vi "Calibrate pH Sensor.vi"(6 "Initialize/Close?":bool, 7 "Calibration Standard":dbl, 8 "Error In (No Error)":errorcluster, 9 "Calibrate":bool=TRUE, 10 "Sensor Address In":string="0", 11 "RS232 Port In":refnum<visa-resource-name>="COM11") -> (0 "Error Out":errorcluster, 1 "Sensor Calibrate Response":bool, 2 "Address Out":string, 3 "RS232 Port Out":refnum<visa-resource-name>)   [LabVIEW 2016]
doc: "Sends an SDI-12 Send Identification Command, and returns the various attributes from the sensor's response.\n\nThe total size by the sensor must be 22-35 in size (inclusive), or this VI will return an error."
uses:
  SDI-12.lvlib
panel:
  out "read buffer":string
  out "output 1":i16
  out "Command":string
  # "(c) 2008 National Instruments.  ALL RIGHTS RESERVED."
  # "The following are required,\nor are optional, for the sensors\nto respond with:"
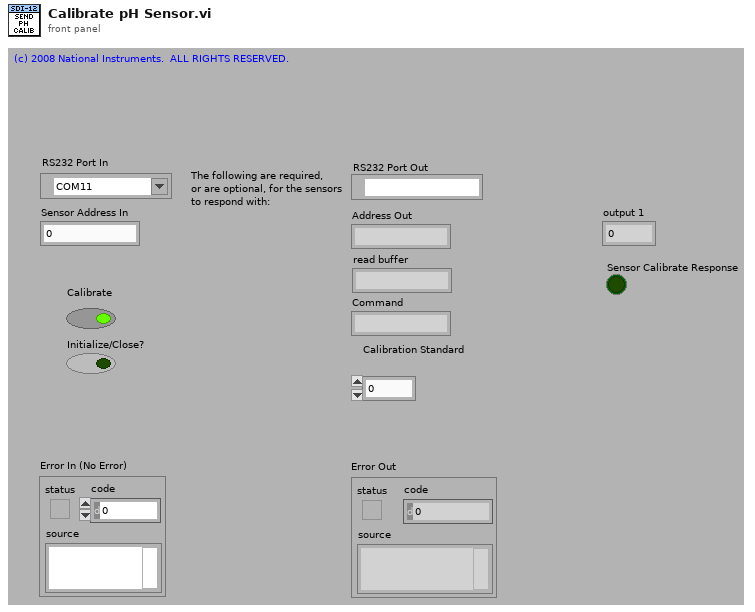
[diagram p1: front panel]
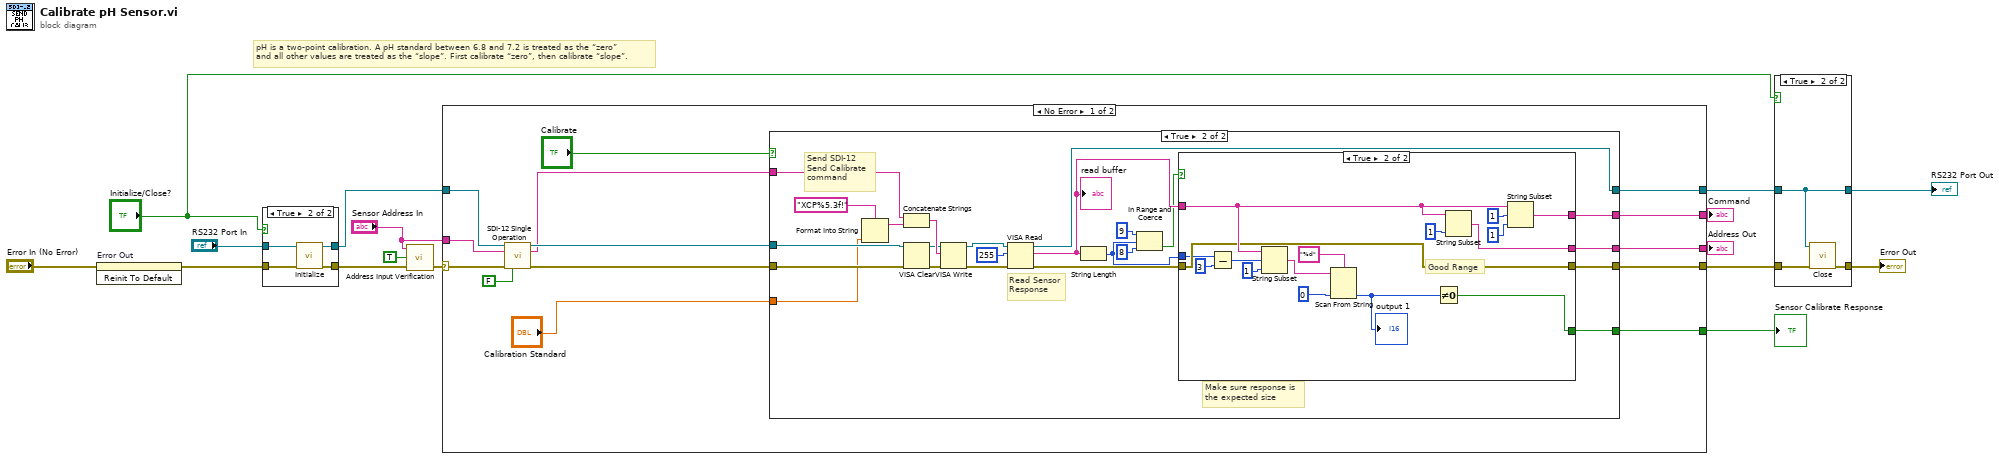
[diagram p0: block diagram]
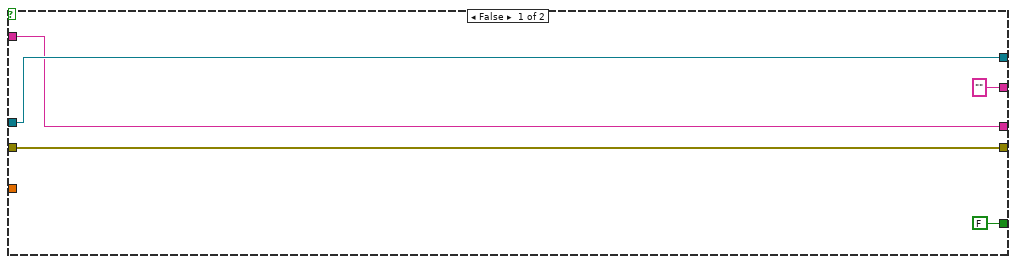
[diagram p4: hidden frame]
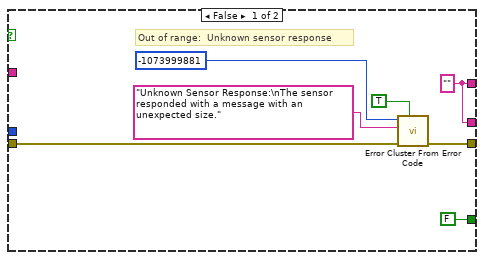
[diagram p5: hidden frame]
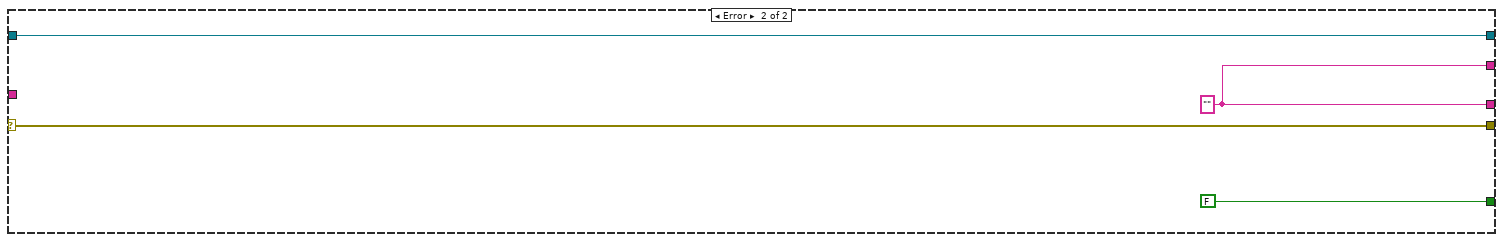
[diagram p6: hidden frame]
diagram:
  # "pH is a two-point calibration. A pH standard between 6.8 and 7.2 is treated as the “zero”\nand all other values are treated as the “slope”. First calibrate “zero”, then calibrate “slope”."
  n1 = invoke on="Error Out" class="Clust (strict)" method="Reinit To Default"(error in="Error In (No Error)") -> (error out=w1:errorcluster)  [unwired: 2 in, 2 out]
  n2 = case shown="True" "Initialize/Close?" {
    tunnel: w1 -> [w18 w22]
    tunnel: [w18 w21] -> w6
    tunnel: "RS232 Port In" -> [w17 w20]
    tunnel: [w17 w19] -> w4
    frame False {
    }
    frame True {
      n3 = call "Initialize.vi"("Error In (No Error)"=w22, "RS232 Port In"=w20) -> ("Error Out"=w21:errorcluster, "RS232 Port Out"=w19:refnum<visa-resource-name>)  [unwired: 8 in]
    }
  }
  n4 = call "Address Input Verification.vi"("Error In (No Error)"=w6, "Error if Bad? (True)"=TRUE ("error if bad? (True)"), "Sensor Address In (a)"="Sensor Address In") -> ("Error Out"=w16:errorcluster)  [unwired: 1 in, 1 out]
  n5 = case shown="No Error" w16 {
    selector: w16 -> [w30 w91]
    tunnel: [w35 w91] -> w10
    tunnel: "Sensor Address In" -> [w26 _]
    tunnel: w4 -> [w28 w90]
    tunnel: [w36 w90] -> w7
    tunnel: [w34 w89] -> w12
    tunnel: [w33 w89] -> w13
    tunnel: [w32 FALSE] -> w11
    frame No Error {
      n6 = call "SDI-12 Single Operation.vi"("RS232 Port In"=w28, "Sensor Address In"=w26, "Error In (No Error)"=w30, "Initialize/Close?"=FALSE) -> ("RS232 Port Out"=w27:refnum<visa-resource-name>, "Address Out"=w25:string, "Error Out"=w29:errorcluster)  [unwired: 7 in, 2 out]
      n7 = case shown="True" "Calibrate" {
        tunnel: w25 -> [w39 w61]
        tunnel: w27 -> [w41 w59]
        tunnel: [w41 w58] -> w36
        tunnel: [w40 w52] -> w35
        tunnel: ["" ("read buffer") w51] -> w34
        tunnel: [w39 w50] -> w33
        tunnel: [FALSE w47] -> w32
        tunnel: w29 -> [w40 w45]
        tunnel: "Calibration Standard" -> [_ w42]
        frame False {
        }
        frame True {
          # "Make sure response is\nthe expected size"
          # "Send SDI-12 \nSend Calibrate \ncommand"
          # "Read Sensor\nResponse"
          n8 = Format Into String(format string="XCP%5.3f!", w42) -> (resulting string=w48:string)  [unwired: 2 in, 1 out]
          n9 = Concatenate Strings(w61, w48) -> (w60:string)
          n10 = VISA Clear(VISA resource name=w59, error in (no error)=w45) -> (VISA resource name out=w46:refnum<visa-resource-name>, error out=w44:errorcluster)
          n11 = VISA Write(VISA resource name=w46, write buffer=w60, error in (no error)=w44) -> (VISA resource name out=w64:refnum<visa-resource-name>, error out=w63:errorcluster)  [unwired: 1 out]
          n12 = VISA Read(VISA resource name=w64, byte count=u32 255, error in (no error)=w63) -> (VISA resource name out=w58:refnum<visa-resource-name>, read buffer=w54:string, error out=w55:errorcluster)  [unwired: 1 out]
          "read buffer" <- w54
          n13 = String Length(string=w54) -> (length=w43:i32)
          n14 = In Range and Coerce(upper limit=9, x=w43, lower limit=8) -> (In Range?=w53:bool)  [unwired: 1 out]
          n15 = case shown="True" w53 {
            tunnel: w55 -> [w67 w82]
            tunnel: [w68 w82] -> w52
            tunnel: w54 -> [_ w84]
            tunnel: [w66 w80] -> w51
            tunnel: [w66 w79] -> w50
            tunnel: [FALSE w75] -> w47
            tunnel: w43 -> [_ w74]
            frame False {
              w66 = "" ("read buffer")
              # "Out of range:  Unknown sensor response"
              n16 = call <vilib>:"Error Cluster From Error Code.vi"("show call chain? (False)"=TRUE, "error in (no error)"=w67, "error message (\"\")"="Unknown Sensor Response:\nThe sensor responded with a message with an unexpected size." ("error message (\"\")"), "error code (0)"=-1073999881) -> ("error out"=w68:errorcluster)  [unwired: 5 in]
            }
            frame True {
              # "Good Range"
              n17 = Subtract(x=w74, y=3) -> (x-y=w73:i32)
              n18 = String Subset(string=w84, offset (0)=w73, length (rest)=1 ("length (rest)")) -> (substring=w81:string)
              n19 = Scan From String(format string="%d", input string=w81, default 1=i16 0 ("default value 1")) -> (output 1=w76:i16)  [unwired: 2 in, 3 out]
              "output 1" <- w76
              n20 = Not Equal To 0?(x=w76) -> (x != 0?=w75:bool)
              n21 = String Subset(string=w84, length (rest)=1 ("length (rest)")) -> (substring=w79:string)  [unwired: 1 in]
              n22 = String Subset(string=w84, offset (0)=1, length (rest)=1 ("length (rest)")) -> (substring=w80:string)
            }
          }
        }
      }
    }
    frame Error {
      w89 = "" ("read buffer")
    }
  }
  "Command" <- w12
  "Address Out" <- w13
  "Sensor Calibrate Response" <- w11
  n23 = case shown="True" "Initialize/Close?" {
    tunnel: w10 -> [w93 w96]
    tunnel: [w93 w95] -> w9
    tunnel: w7 -> [w92 w94]
    tunnel: [w92 w94] -> w8
    frame False {
    }
    frame True {
      n24 = call "Close.vi"("Error In (No Error)"=w96, "RS232 Port In"=w94) -> ("Error Out"=w95:errorcluster)  [unwired: 9 in]
    }
  }
  "Error Out" <- w9
  "RS232 Port Out" <- w8
